vi "datalogger_1.vi"() -> ()   [LabVIEW 2015]
uses:
  <vilib>/Utility/file.llb/Write Delimited Spreadsheet (string).vi
  <vilib>/Utility/file.llb/Write Delimited Spreadsheet (DBL).vi
panel:
  out "appended array":dbl[][](array[numeric]) format="%#.3g"
  in  "file path (dialog if empty)":path
  out "Array":string[](array[string])
  in  "stop":bool
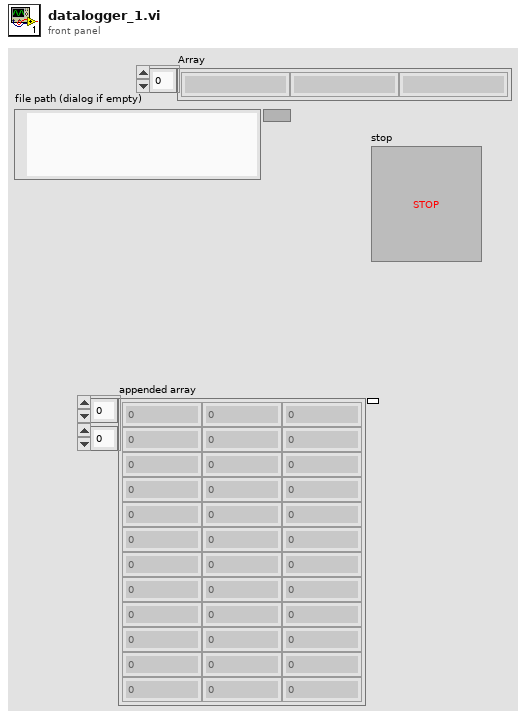
[diagram p1: front panel]
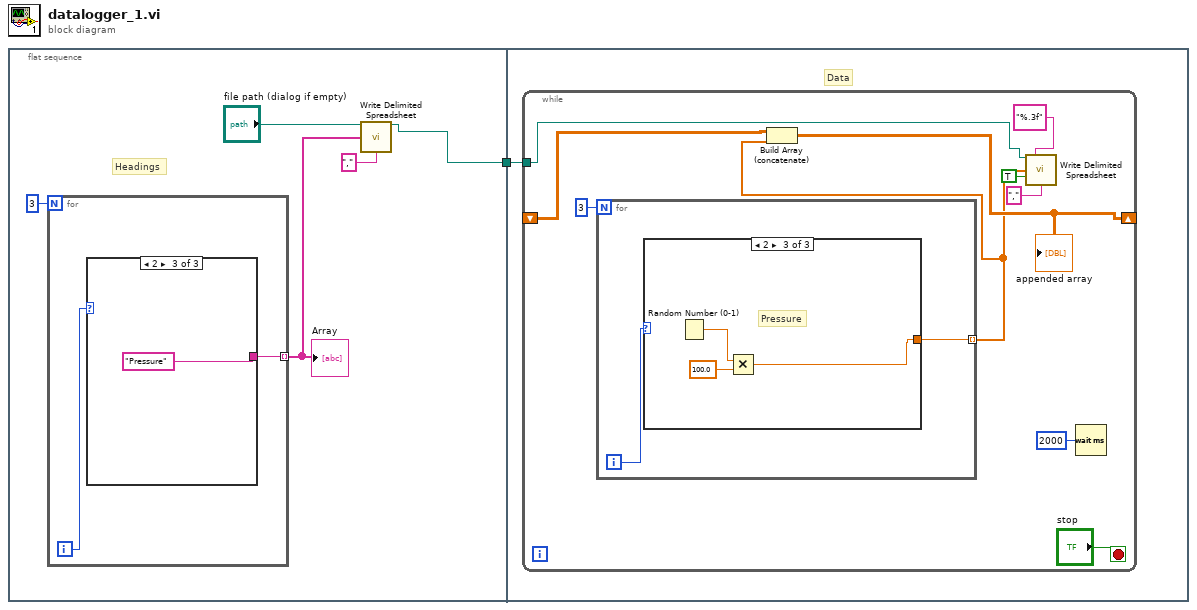
[diagram p0: block diagram]
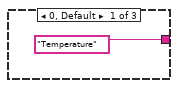
[diagram p2: hidden frame]
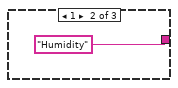
[diagram p3: hidden frame]
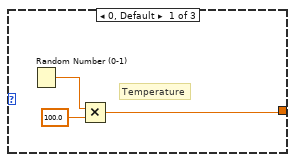
[diagram p4: hidden frame]
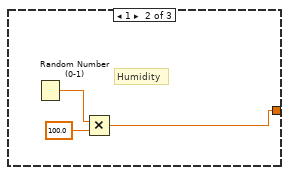
[diagram p5: hidden frame]
diagram:
  n1 = flat-sequence {
    tunnel: [w2] -> w1
    tunnel: w1 -> [w12]
    frame #0 {
      # "Headings"
      n2 = for {
        N: 3 -> [_]
        tunnel: [w7] -> w4 mode=indexing
        i -> [w8]
        n3 = case shown="2" w8 {
          tunnel: ["Temperature" "Humidity" "Pressure"] -> w7
          frame 0, Default {
          }
          frame 1 {
          }
          frame 2 {
          }
        }
      }
      "Array" <- w4
      n4 = call-poly <vilib>:"Write Delimited Spreadsheet.vi"("file path (dialog if empty)"="file path (dialog if empty)", "1D data"=w4, "delimiter (\\t)"="," ("delimiter (\\t)")) -> ("new file path (Not A Path if cancelled)"=w2:path)  [unwired: 11 in, 1 out]
    }
    frame #1 {
      # "Data"
      n5 = while {
        tunnel: w12 -> [w13]
        shift-right: [w16] -> _
        shift-left: _ -> [w17]
        stop <- "stop" stop-if-true
        n6 = for {
          N: 3 -> [_]
          tunnel: [w23] -> w15 mode=indexing
          i -> [w24]
          n7 = case shown="2" w24 {
            tunnel: [w25 w28 w31] -> w23
            frame 0, Default {
              # "Temperature"
              n8 = Random Number (0-1)() -> (number: 0 to 1=w27:dbl)
              n9 = Multiply(x=w27, y=100.0) -> (x*y=w25:dbl)
            }
            frame 1 {
              # "Humidity"
              n10 = Random Number (0-1)() -> (number: 0 to 1=w29:dbl)
              n11 = Multiply(x=w29, y=100.0) -> (x*y=w28:dbl)
            }
            frame 2 {
              # "Pressure"
              n12 = Random Number (0-1)() -> (number: 0 to 1=w32:dbl)
              n13 = Multiply(x=w32, y=100.0) -> (x*y=w31:dbl)
            }
          }
        }
        n14 = Build Array (concatenate)(w17, w15) -> (w16:dbl[][])
        "appended array" <- w16
        n15 = call-poly <vilib>:"Write Delimited Spreadsheet.vi"("file path (dialog if empty)"=w13, "format (%.3f)"="%.3f", "1D data"=w15, "append to file? (F)"=TRUE, "delimiter (\\t)"="," ("delimiter (\\t)")) -> ()  [unwired: 9 in, 2 out]
        n16 = Wait (ms)(milliseconds to wait=u32 2000) -> ()  [unwired: 1 out]
      }
    }
  }
